vi "Extension Setpoint.vi"() -> (1 "Setpoint":dbl, 2 "Axis 4":dbl)   [LabVIEW 2011]
uses:
  Robot Global Data.vi
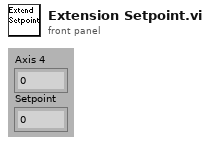
[diagram p1: front panel]
types:
  T1 = cluster{"Axis 1":dbl, "Axis 2":dbl, "Axis 3":dbl, "Axis 4":dbl, "Axis 5":dbl, "Axis 6":dbl, "Button 1":bool, "Button 2":bool, "Button 3":bool, "Button 4":bool, "Button 5":bool, "Button 6":bool, "Button 7":bool, "Button 8":bool, "Button 9":bool, "Button 10":bool, "Button 11":bool, "Button 12":bool}
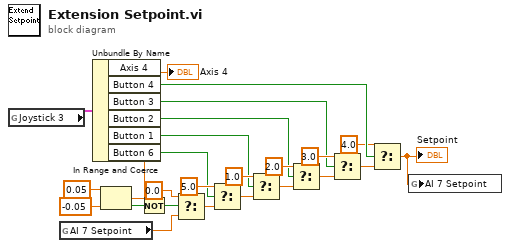
[diagram p0: block diagram]
diagram:
  n1 = global read "Robot Global Data.vi" "Joystick 3"() -> (w24:T1)
  n2 = global read "Robot Global Data.vi" "AI 7 Setpoint"() -> (w2:dbl)
  n3 = Unbundle By Name(w24) -> ("Axis 4"=w8:dbl, "Button 4"=w13:bool, "Button 3"=w12:bool, "Button 2"=w14:bool, "Button 1"=w15:bool, "Button 6"=w10:bool)
  "Axis 4" <- w8
  n4 = In Range and Coerce(upper limit=0.05, x=w8, lower limit=-0.05) -> (In Range?=w9:bool)  [unwired: 1 out]
  n5 = Not(x=w9) -> (.not. x?=w4:bool)
  n6 = Select(t=0.0, s=w4, f=w2) -> (s? t:f=w5:dbl)
  n7 = Select(t=5.0, s=w10, f=w5) -> (s? t:f=w16:dbl)
  n8 = Select(t=1.0, s=w15, f=w16) -> (s? t:f=w22:dbl)
  n9 = Select(t=2.0, s=w14, f=w22) -> (s? t:f=w21:dbl)
  n10 = Select(t=3.0, s=w12, f=w21) -> (s? t:f=w20:dbl)
  n11 = Select(t=4.0, s=w13, f=w20) -> (s? t:f=w1:dbl)
  "Setpoint" <- w1
  n12 = global write "Robot Global Data.vi" "AI 7 Setpoint"(w1) -> ()
